vi "Ex3_Chaine_de_caractere.vi"() -> ()   [LabVIEW 2018]
panel:
  out "ERREUR":bool
  out "Nom":string
  out "Prénom":string
  in  "Nom Brut":string
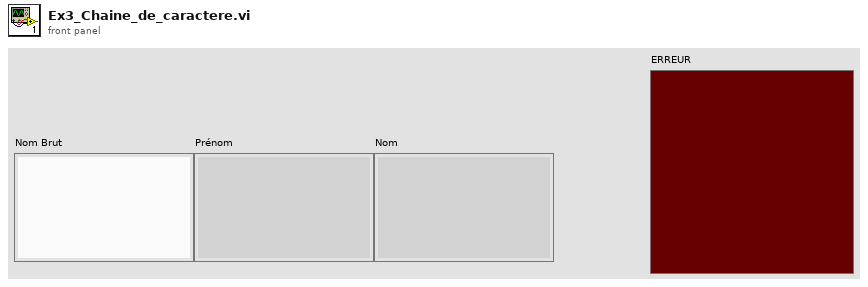
[diagram p1: front panel]
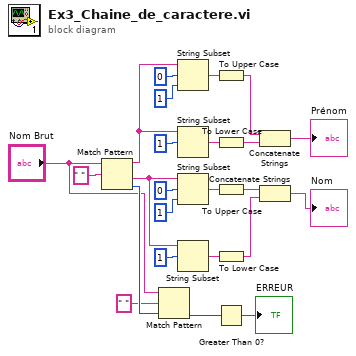
[diagram p0: block diagram]
diagram:
  n1 = Match Pattern(string="Nom Brut", regular expression=" ") -> (before substring=w14:string, after substring=w1:string, offset past match=w23:i32)  [unwired: 1 in, 1 out]
  n2 = Match Pattern(string="Nom Brut", regular expression=" " ("string"), offset (0)=w23) -> (offset past match=w20:i32)  [unwired: 3 out]
  n3 = String Subset(string=w14, offset (0)=0, length (rest)=1 ("length (rest)")) -> (substring=w16:string)
  n4 = String Subset(string=w14, offset (0)=1) -> (substring=w13:string)  [unwired: 1 in]
  n5 = String Subset(string=w1, offset (0)=0, length (rest)=1 ("length (rest)")) -> (substring=w7:string)
  n6 = String Subset(string=w1, offset (0)=1) -> (substring=w5:string)  [unwired: 1 in]
  n7 = To Upper Case(1:w16) -> (0:w12:string)
  n8 = To Lower Case(string=w13) -> (all lower case string=w11:string)
  n9 = To Upper Case(1:w7) -> (0:w4:string)
  n10 = To Lower Case(string=w5) -> (all lower case string=w3:string)
  n11 = Greater Than 0?(x=w20) -> (x > 0?=→"ERREUR":bool)
  n12 = Concatenate Strings(w12, w11) -> (→"Prénom":string)
  n13 = Concatenate Strings(w4, w3) -> (→"Nom":string)
